vi "Test - Draw Textured Triangle.vi"() -> ()   [LabVIEW 2022 SP3, in "Raster.lvlib"]
uses:
  Raster.lvlib
  Point 2D.ctl
  UV.ctl
  Rectangle Dimensions.ctl
  5ea285c7-be76-47ab-bb95-511c6a9aac96.vi
  d84cddbd-8e40-43c7-a758-6e8d8fd6f2c6.vi
  <vilib>/Utility/High Resolution Relative Seconds.vi
  Utility/Convert Pixels To Picture.vi/d601d993-a776-4dc8-89c7-357d8398c88c.vi
  Utility/Convert Pixels To Picture.vi/7816d0d6-8e4d-41a2-85ac-ed82f1435763.vi
  <vilib>/picture/picture.llb/Draw Unflattened Pixmap.vi
  <vilib>/picture/picture.llb/Draw True-Color Pixmap.vi
  Utility/Utility.lvlib
panel:
  in  "Texture 3":T1={"u"=0.814, "v"=0.357} {"v" min=0 max=1 step=0.1; "u" min=0 max=1 step=0.1}
  in  "Point 3":T2={"x"=90, "y"=303}
  in  "Texture 2":T1={"u"=0.317, "v"=0.766} {"v" min=0 max=1 step=0.1; "u" min=0 max=1 step=0.1}
  in  "Point 2":T2={"x"=390, "y"=98}
  in  "Texture 1":T1={"u"=0.739, "v"=0.913} {"v" min=0 max=1 step=0.1; "u" min=0 max=1 step=0.1}
  in  "Point 1":T2={"x"=49, "y"=26}
  out "Time [s]":dbl format="%.3p"
  out "new picture":picture
  # "(0,0)"
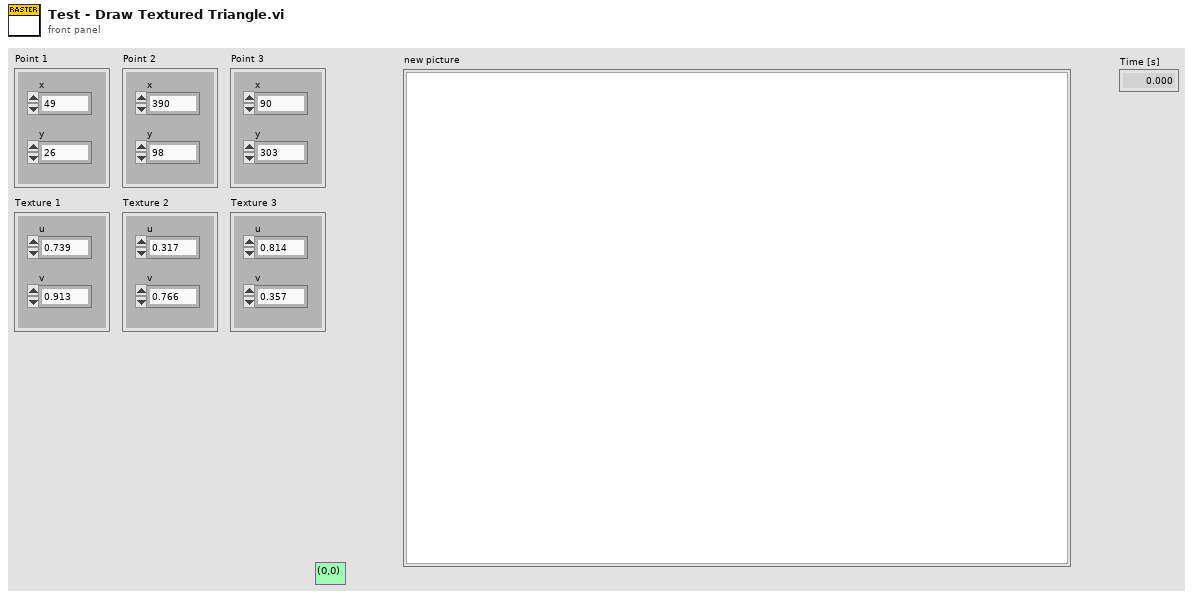
[diagram p1: front panel]
types:
  T1 = typedef "Raster.lvlib/UV.ctl" = cluster{"u":sgl, "v":sgl}
  T2 = typedef "Raster.lvlib/Point 2D.ctl" = cluster{"x":i32, "y":i32}
  T3 = typedef "Raster.lvlib/Rectangle Dimensions.ctl" = cluster{"Width":u32, "Height":u32}
  T4 = typedef "imagedata.ctl" = cluster{"image type":i32, "image depth":i32, "image":u8[], "mask":u8[], "colors":u32[], "Rectangle":cluster{"left":i16, "top":i16, "right":i16, "bottom":i16}}
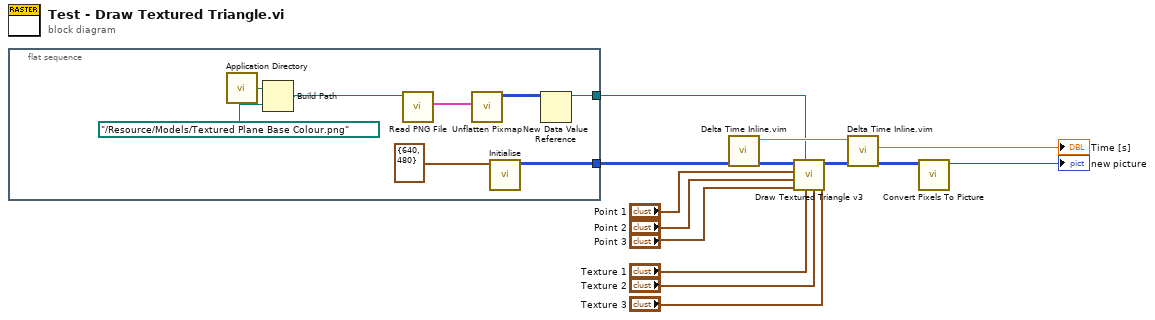
[diagram p0: block diagram]
diagram:
  n1 = flat-sequence {
    tunnel: [w21] -> w13
    tunnel: [w18] -> w1
    frame #0 {
      n2 = call <vilib>:"Application Directory.vi"() -> ("Application Directory"=w16:path)
      n3 = Build Path(base path=w16, name or relative path=path "../Resource/Models/Textured Plane Base Colour.png") -> (appended path=w15:path)
      n4 = call <vilib>:"Read PNG File.vi"("path to PNG file"=w15) -> ("image data"=w20:T4)  [unwired: 8 in, 2 out]
      n5 = call <vilib>:"Unflatten Pixmap.vi"("image data"=w20) -> ("24-bit pixmap"=w19:u32[][])  [unwired: 4 in, 6 out]
      n6 = call "Initialise.vi"("Screen Dimensions"=T3 {"Width"=640, "Height"=480}) -> ("Pixel Data out"=w21:u32[][])  [unwired: 10 in]
      n7 = New Data Value Reference(data value=w19) -> (data value reference=w18:refnum<data-value>)  [unwired: 1 in, 1 out]
    }
  }
  n8 = call "Delta Time Inline.vim"("value in"=w13) -> ("value out"=w9:u32[][], "Relative Seconds out [s]"=w10:dbl)  [unwired: 8 in, 1 out]
  n9 = call "Draw Textured Triangle v3.vi"("Texture 3"="Texture 3", "Texture 2"="Texture 2", "Texture 1"="Texture 1", "Texture"=w1, "Point 3"="Point 3", "Point 2"="Point 2", "Point 1"="Point 1", "Pixel Data in"=w9) -> ("Pixel Data out"=w8:u32[][])  [unwired: 3 in]
  n10 = call "Delta Time Inline.vim"("value in"=w8, "Relative Seconds in [s]"=w10) -> ("value out"=w12:u32[][], "Delta Time [s]"=→"Time [s]":dbl)  [unwired: 7 in, 1 out]
  n11 = call "Convert Pixels To Picture.vi"("Pixel Data in"=w12) -> ("2D Picture"=→"new picture":picture)  [unwired: 9 in, 1 out]
